vi "Get command-data.vi"(8 "error in (no error)":errorcluster, 11 "Message Response in":refnum<class "Message Response.lvclass">) -> (0 "error out":errorcluster, 1 "Cluster":T1, 2 "Name":string, 3 "Message Response out":refnum<class "Message Response.lvclass">)   [LabVIEW 2016, in "WebSocket Networking.lvlib" / "Message Response.lvclass"]
uses:
  <userlib>/Common Components/WebSocket Networking/Message Response/Message Response.lvclass
  C:/Program Files (x86)/National Instruments/LabVIEW 2016/user.lib/Composed Systems/Stream/Mediator/Classes/Message Interface/Message Interface.lvclass
  <userlib>/Common Components/Common/command-data.ctl
  <userlib>/Common Components/WebSocket Networking/Message Response/Message Response.lvclass/Message Response.ctl
  <userlib>/Composed Systems/Stream/Mediator/Classes/Message Interface/Message Interface.lvclass
  <userlib>/Common Components/Common/Common.lvlib
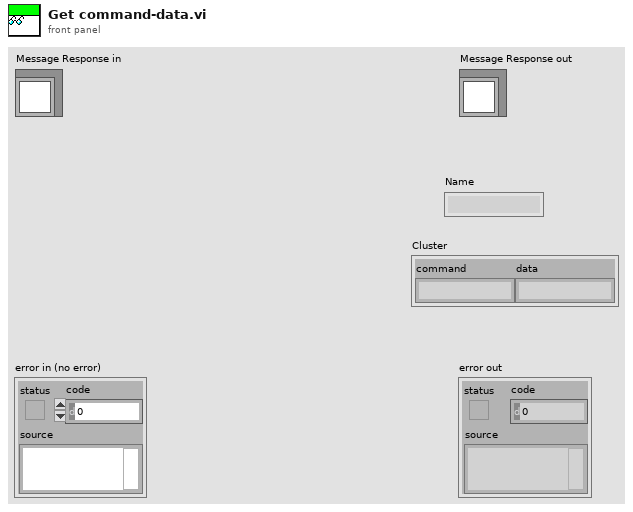
[diagram p1: front panel]
types:
  T1 = typedef "Common.lvlib/command-data.ctl" = cluster{"command":string, "data":string}
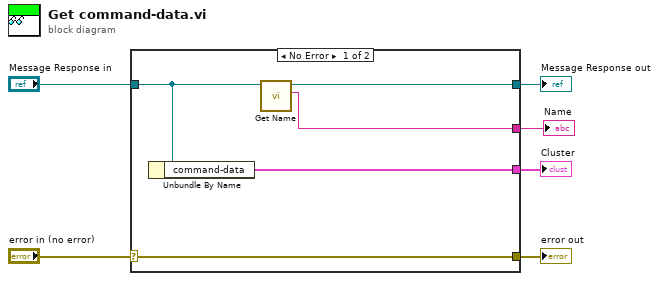
[diagram p0: block diagram]
diagram:
  n1 = case shown="No Error" "error in (no error)" {
    selector: "error in (no error)" -> [w11 w12]
    tunnel: [w11 w12] -> w5
    tunnel: [w8 w13] -> w3
    tunnel: "Message Response in" -> [w9 w13]
    tunnel: [w10 _] -> w2
    tunnel: [w7 _] -> w1
    frame No Error {
      n2 = Unbundle By Name(w9) -> ("command-data"=w10:T1)
      n3 = call <userlib>:"Get Name.vi"("Message Interface in"=w9) -> ("Name"=w7:string, "Message Interface out"=w8:refnum<class "Message Response.lvclass">)  [unwired: 8 in, 1 out]
    }
    frame Error {
    }
  }
  "error out" <- w5
  "Message Response out" <- w3
  "Cluster" <- w2
  "Name" <- w1
